vi "Escribir TDMS Parametro del Generador.vi"(7 "semaphore":T1, 8 "error in (no error)":errorcluster, 9 "queue":refnum<queue>) -> (0 "error out":errorcluster, 1 "queue out":refnum<queue>, 2 "tdms sinc out":refnum<k34>, 3 "tdms historico out":refnum<k34>, 5 "semaphore out":T1)   [LabVIEW 2015]
uses:
  ClusterM2.ctl
panel:
  out "M2":T2
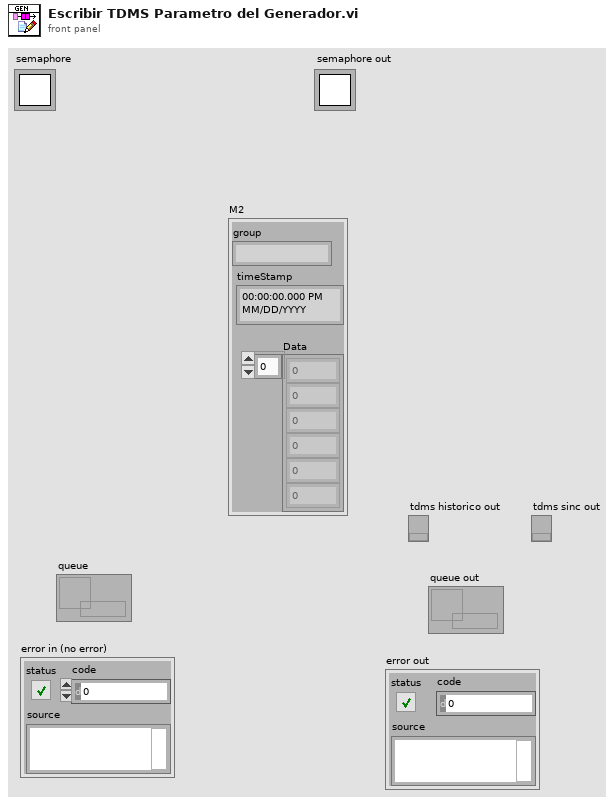
[diagram p1: front panel]
types:
  T1 = typedef "Semaphore RefNum" = refnum<k1>
  T2 = typedef "ClusterM2.ctl" = cluster{"timeStamp":timestamp, "Data":dbl[], "group":string}
  T3 = cluster{"tdms control out":refnum<k34>, "tdms historial out":refnum<k34>, "tdms sinc out":refnum<k34>}
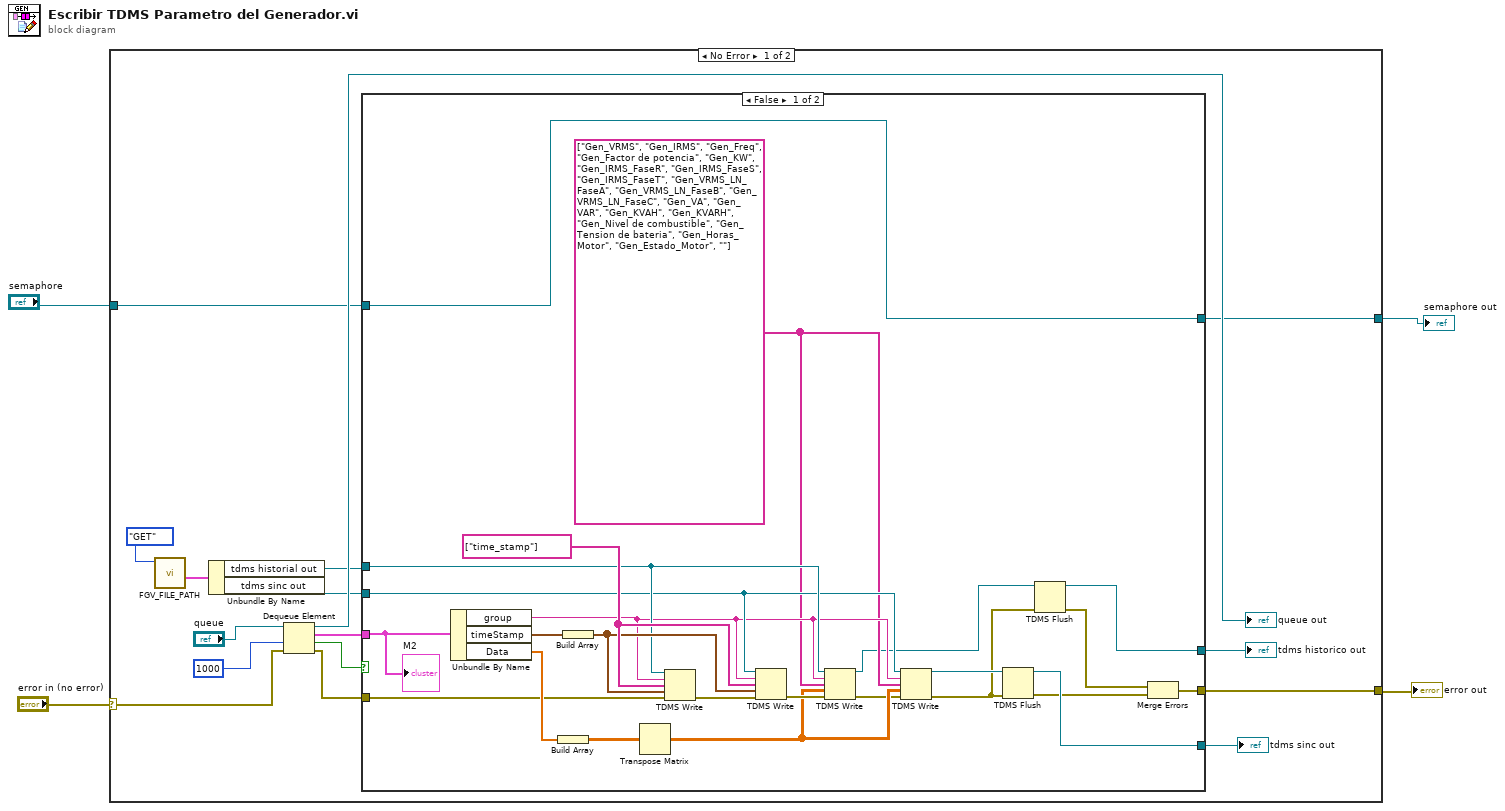
[diagram p0: block diagram]
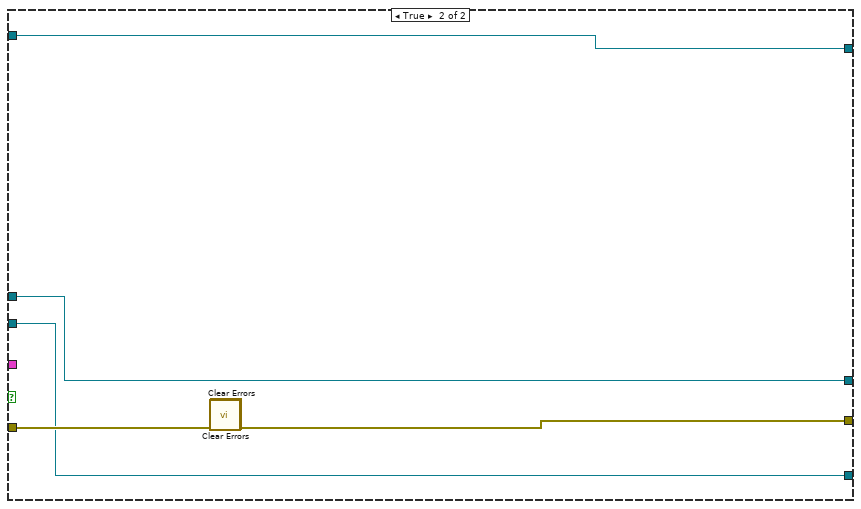
[diagram p2: hidden frame]
diagram:
  n1 = case shown="No Error" "error in (no error)" {
    selector: "error in (no error)" -> [w8 w51]
    tunnel: [w7 w51] -> w3
    tunnel: "semaphore" -> [w6 w50]
    tunnel: [w5 w50] -> w1
    frame No Error {
      n2 = call "FGV_FILE_PATH.vi"("Function"=enum16{"GET", "SET"}."GET") -> ("Data Out"=w11:T3)  [unwired: 10 in]
      n3 = Unbundle By Name(w11) -> ("tdms historial out"=w10:refnum<k34>, "tdms sinc out"=w9:refnum<k34>)
      n4 = Dequeue Element(queue="queue", timeout in ms (-1)=1000, error in (no error)=w8) -> (queue out=→"queue out":refnum<queue>, element=w19:T2, timed out?=w20:bool, error out=w15:errorcluster)
      n5 = case shown="False" w20 {
        tunnel: w19 -> [w43 _]
        tunnel: w15 -> [w36 w49]
        tunnel: [w24 w48] -> w7
        tunnel: w10 -> [w37 w47]
        tunnel: w9 -> [w34 w46]
        tunnel: [w27 w47] -> w14
        tunnel: [w25 w46] -> w13
        tunnel: [w29 w45] -> w5
        tunnel: w6 -> [w29 w45]
        frame False {
          w32 = string[] ["Gen_VRMS", "Gen_IRMS", "Gen_Freq", "Gen_Factor de potencia", "Gen_KW", "Gen_IRMS_FaseR", "Gen_IRMS_FaseS", "Gen_IRMS_FaseT", "Gen_VRMS_LN_FaseA", "Gen_VRMS_LN_FaseB", "Gen_VRMS_LN_FaseC", "Gen_VA", "Gen_VAR", "Gen_KVAH", "Gen_KVARH", "Gen_Nivel de combustible", "Gen_Tension de bateria", "Gen_Horas_Motor", "Gen_Estado_Motor", ""]
          w40 = string[] ["time_stamp"] ("channel name(s) in (Untitled)")
          n6 = Unbundle By Name(w43) -> ("group"=w33:string, "timeStamp"=w44:timestamp, "Data"=w42:dbl[])
          n7 = Build Array(w42) -> (w41:dbl[][])
          n8 = Build Array(w44) -> (w39:timestamp[])
          n9 = Transpose Matrix(1:w41) -> (0:w31:dbl[][])
          n10 = TDMS Write(0:w37, 5:w33, 7:w40, 9:w39, 11:w36) -> (15:w38:errorcluster)  [unwired: 1 in, 3 out]
          n11 = TDMS Write(0:w34, 5:w33, 7:w40, 9:w39, 11:w38) -> (15:w35:errorcluster)  [unwired: 1 in, 3 out]
          n12 = TDMS Write(0:w37, 5:w33, 7:w32, 9:w31, 11:w35) -> (4:w28:refnum<k34>, 15:w30:errorcluster)  [unwired: 1 in, 2 out]
          n13 = TDMS Write(0:w34, 5:w33, 7:w32, 9:w31, 11:w30) -> (4:w26:refnum<k34>, 15:w23:errorcluster)  [unwired: 1 in, 2 out]
          n14 = TDMS Flush(4:w23, 7:w26) -> (0:w22:errorcluster, 3:w25:refnum<k34>)
          n15 = TDMS Flush(4:w23, 7:w28) -> (0:w21:errorcluster, 3:w27:refnum<k34>)
          n16 = Merge Errors(w21, w22) -> (w24:errorcluster)
          "M2" <- w43
        }
        frame True {
          n17 = call <vilib>:"Clear Errors.vi"("error in (no error)"=w49) -> ("error out"=w48:errorcluster)  [unwired: 5 in, 1 out]
          n18 = call <vilib>:"Clear Errors.vi"() -> ()  [unwired: 6 in, 2 out]
        }
      }
      "tdms sinc out" <- w13
      "tdms historico out" <- w14
    }
    frame Error {
    }
  }
  "error out" <- w3
  "semaphore out" <- w1
